vi "SDSU_DACS.vi"(0 "refnum":i32, 5 "Command":string, 7 "physical unit":string, 9 "swhitches":string[](array[string]), 11 "error in (no error)":errorcluster, 12 "switch arguments":string[](array[string])) -> (4 "refnum out":i32, 6 "response":string, 15 "error out":errorcluster)   [LabVIEW 2016]
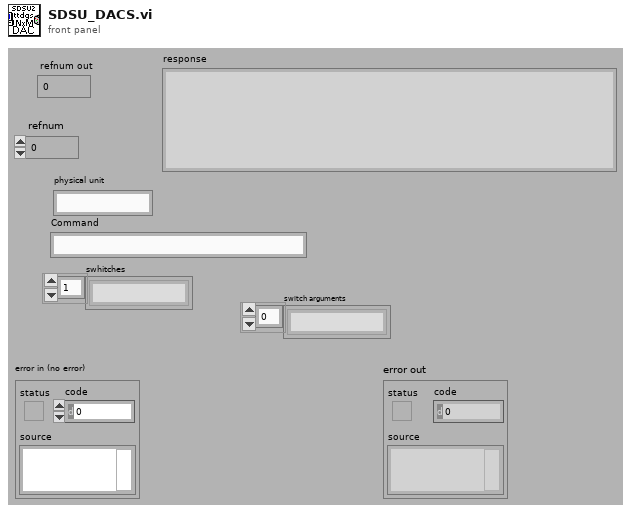
[diagram p1: front panel]
types:
  T1 = enum16{"read from file", "find", "set", "set_to_default", "get all"}
  T2 = enum16{"read from file", "find", "set", "set_to_default"}
  T3 = enum16{"read from file", "find", "set", "set_to_default", "get all", "resend_last"}
  T4 = typedef "CMN_ContStatus.ctl" = cluster{"Response":string, "power":bool, "shutter":bool, "artifdata":bool, "idlemode":bool, "reset":bool, "gain":u8, "speed":u8, "resetPCI":bool, "autoshutter":bool, "TempSetPoint":i32, "multipleextensions":bool, "displayImage":bool, "coadding":bool, "images being coadded":i32, "Operation Mode":enum16{"normal", "coadd", "fawler"}, "frames to write":cluster{"subs":bool, "reset":bool, "exposed":bool}, "fawler samples":i32, "write auto":bool, "datatype":string, "frames to display":cluster{"subs":bool, "reset":bool, "exposed":bool}, "sur":i32, "autoclear":bool}
  T5 = enum16{"Idle", "Exposing", "Paused", "AbortExp", "Reading", "AbortRead", "FinishedReading", "Resetting", "Reducing", "Initializing"}
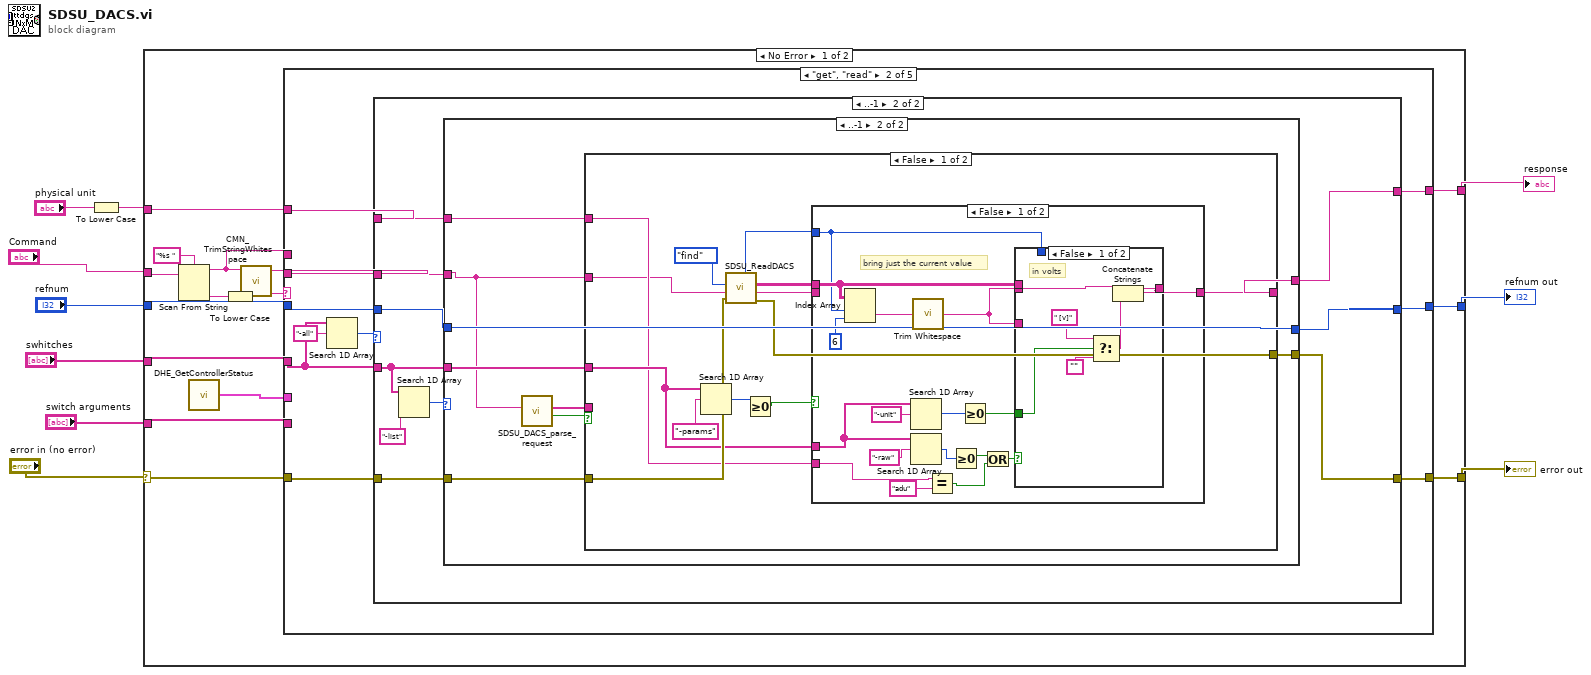
[diagram p0: block diagram]
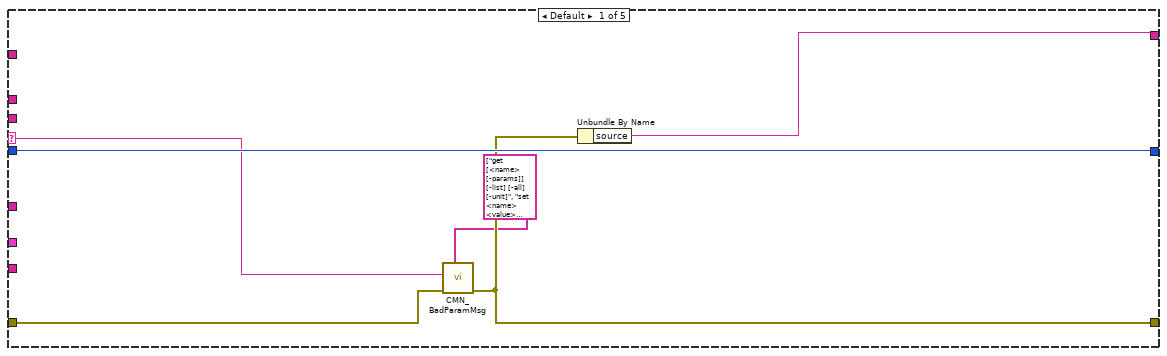
[diagram p2: hidden frame]
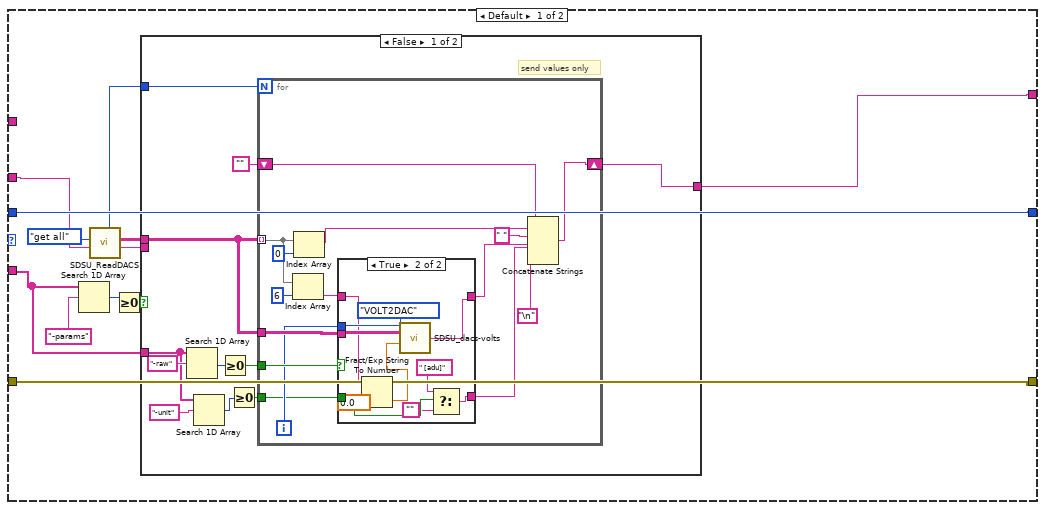
[diagram p3: hidden frame]
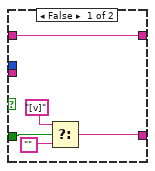
[diagram p4: hidden frame]
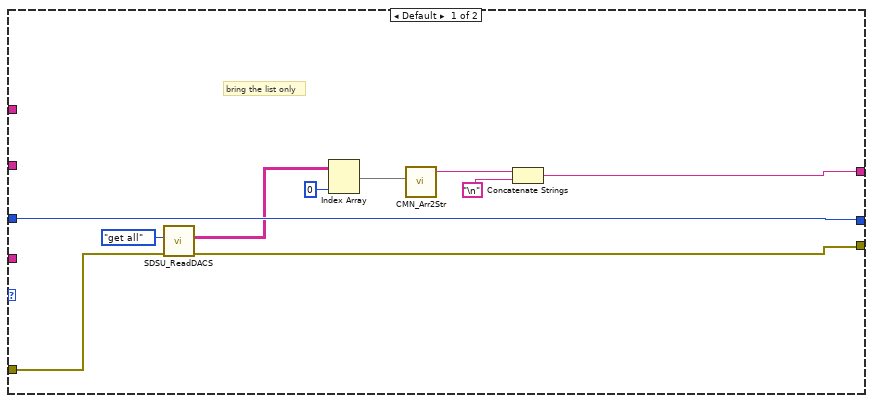
[diagram p6: hidden frame]
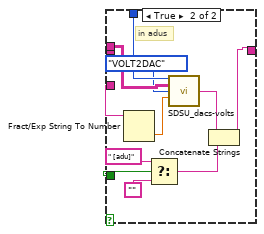
[diagram p7: hidden frame]
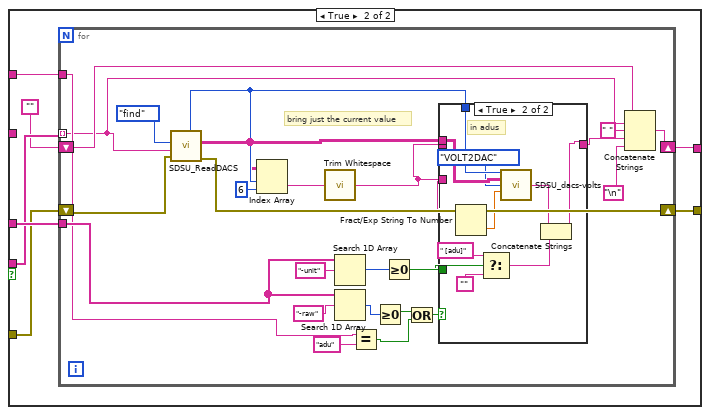
[diagram p9: hidden frame]
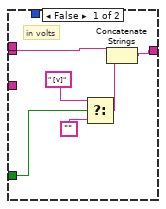
[diagram p10: hidden frame]
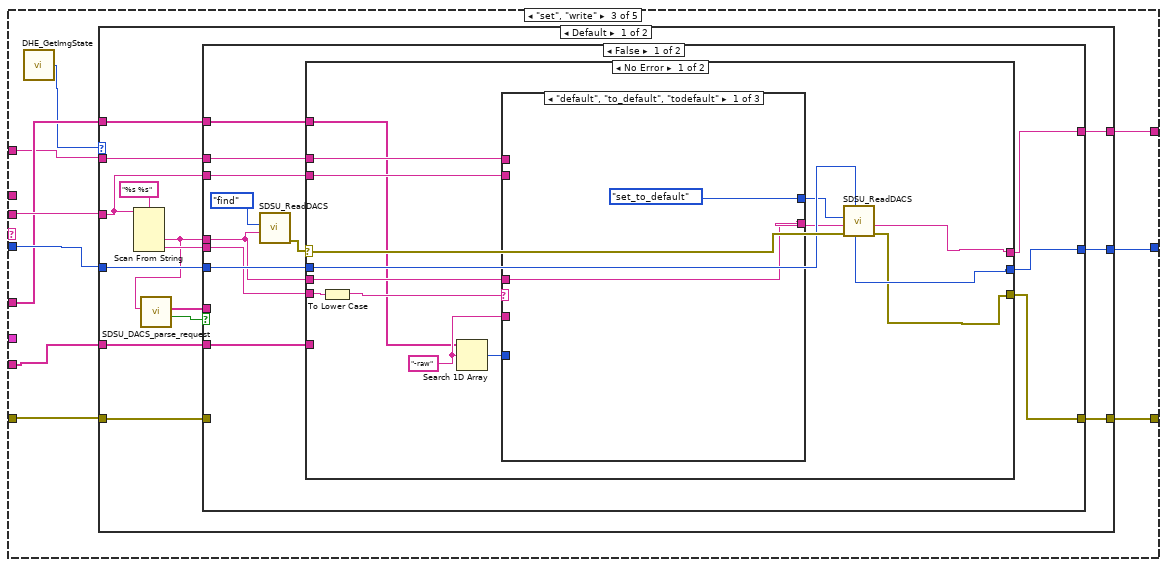
[diagram p11: hidden frame]
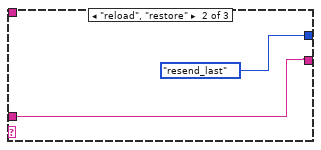
[diagram p12: hidden frame]
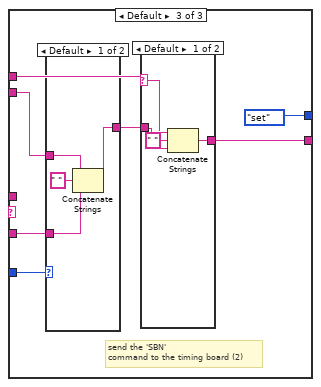
[diagram p13: hidden frame]
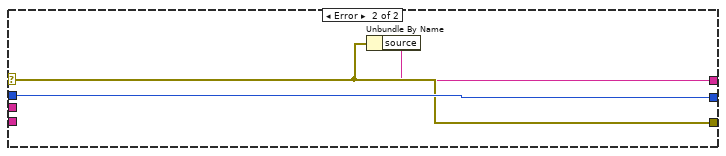
[diagram p16: hidden frame]
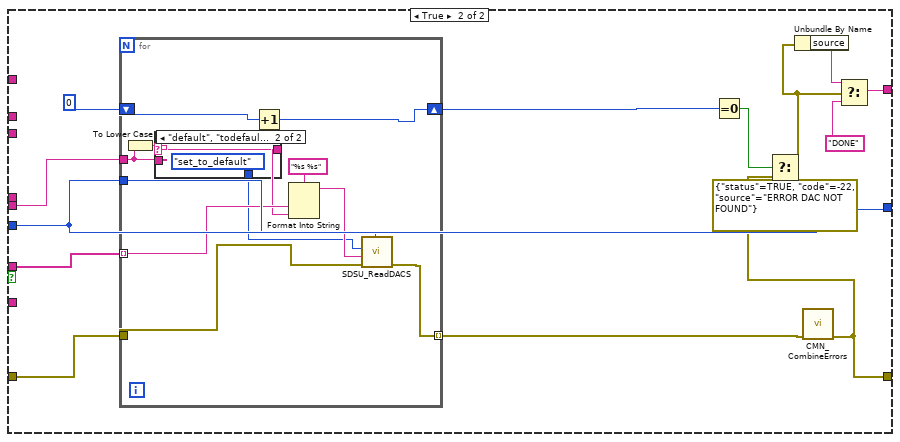
[diagram p17: hidden frame]
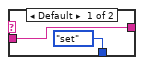
[diagram p18: hidden frame]
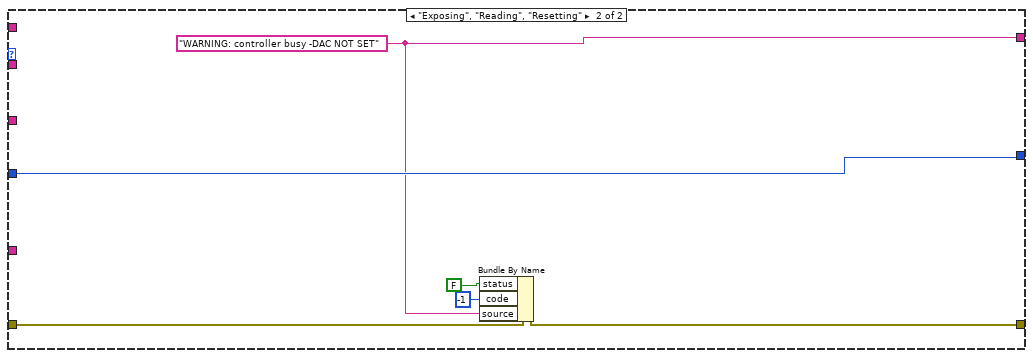
[diagram p19: hidden frame]
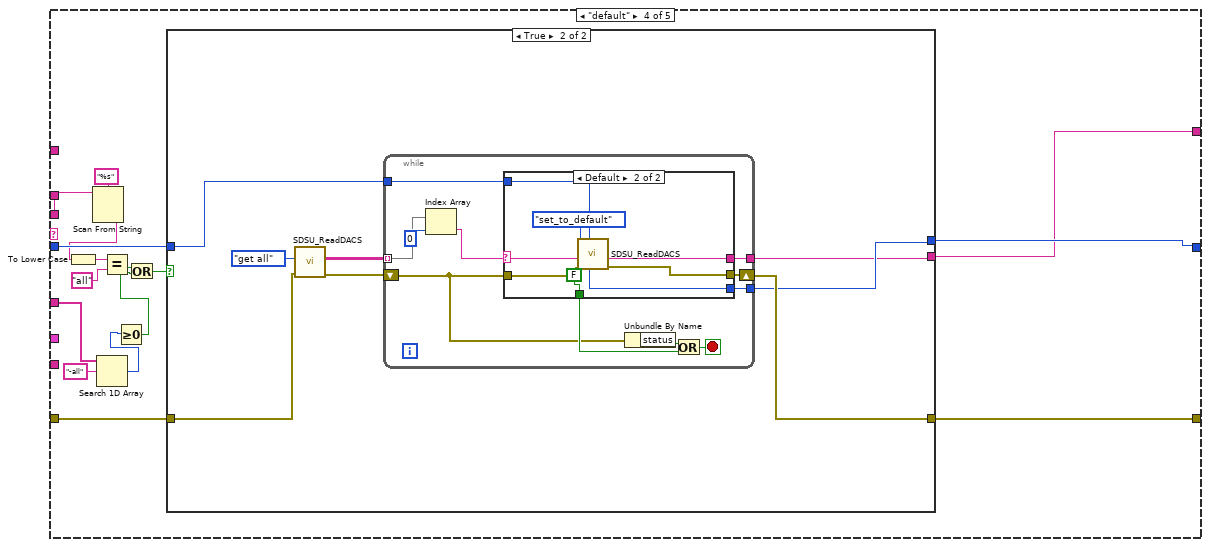
[diagram p20: hidden frame]
diagram:
  n1 = To Lower Case(string="physical unit") -> (all lower case string=w5:string)
  n2 = case shown="No Error" "error in (no error)" {
    selector: "error in (no error)" -> [w12 w440]
    tunnel: [w25 w440] -> w8
    tunnel: "refnum" -> [w24 w442]
    tunnel: [w23 w442] -> w10
    tunnel: "Command" -> [w16 _]
    tunnel: w5 -> [w15 _]
    tunnel: [w14 w441] -> w4
    tunnel: "swhitches" -> [w13 _]
    tunnel: "switch arguments" -> [w11 _]
    frame No Error {
      n3 = Scan From String(format string="%s " ("Format String"), input string=w16) -> (remaining string=w18:string, output 1=w19:string)  [unwired: 2 in, 3 out]
      n4 = call "DHE_GetControllerStatus.vi"() -> ("ControllerStatus"=w17:T4)  [unwired: 11 out]
      n5 = To Lower Case(string=w19) -> (all lower case string=w20:string)
      n6 = call "CMN_TrimStringWhitespace.vi"("string"=w18) -> ("trimmed string"=w21:string)  [unwired: 1 in, 8 out]
      n7 = case shown="\"get\", \"read\"" w20 {
        selector: w20 -> [w29 _ _ _ _]
        tunnel: w12 -> [w30 w36 w231 w338 w391]
        tunnel: [w28 w35 w229 w337 w390] -> w25
        tunnel: w24 -> [w31 w37 w227 w349 w402]
        tunnel: [w31 w41 w230 w336 w389] -> w23
        tunnel: w21 -> [_ w38 w232 w344 w397]
        tunnel: w17 -> [_ _ _ _ _]
        tunnel: w18 -> [_ _ _ _ _]
        tunnel: w15 -> [_ w39 w225 _ _]
        tunnel: [w27 w40 w228 w335 w388] -> w14
        tunnel: w13 -> [_ w34 w226 w334 w387]
        tunnel: w11 -> [_ _ w224 _ _]
        frame Default {
          n8 = call "CMN_BadParamMsg.vi"("valid params"=string[] ["get [<name> [-params]] [-list] [-all] [-unit]", "set <name> <value> [-raw] [default]", "default [-all]"], "error in (no error)"=w30, "parameter"=w29) -> ("error out"=w28:errorcluster)  [unwired: 1 in, 7 out]
          n9 = Unbundle By Name(w28) -> ("source"=w27:string)
        }
        frame "get", "read" {
          n10 = Search 1D Array(1D array=w34, element="-all") -> (index of element=w32:i32)  [unwired: 1 out]
          n11 = case shown="..-1" w32 {
            tunnel: [w50 w106] -> w41
            tunnel: [w51 w105] -> w40
            tunnel: w39 -> [_ w104]
            tunnel: w38 -> [w48 w103]
            tunnel: w37 -> [w50 w102]
            tunnel: w34 -> [w42 w99]
            tunnel: w36 -> [w43 w101]
            tunnel: [w43 w100] -> w35
            frame Default {
              n12 = Search 1D Array(1D array=w42, element="-params") -> (index of element=w52:i32)  [unwired: 1 out]
              n13 = call "SDSU_ReadDACS.vi"("argument"=w48, "action"=T1."get all") -> ("response"=w46:string, "Table"=w45:string[][], "index"=w44:i32)  [unwired: 3 in, 4 out]
              n14 = Greater Or Equal To 0?(x=w52) -> (x >= 0?=w47:bool)
              n15 = case shown="False" w47 {
                tunnel: [w62 w96] -> w51
                tunnel: w46 -> [_ w96]
                tunnel: w45 -> [w58 _]
                tunnel: w44 -> [w64 _]
                tunnel: w42 -> [w57 _]
                frame False {
                  # "send values only"
                  n16 = Search 1D Array(1D array=w57, element="-raw") -> (index of element=w60:i32)  [unwired: 1 out]
                  n17 = Search 1D Array(1D array=w57, element="-unit") -> (index of element=w55:i32)  [unwired: 1 out]
                  n18 = Greater Or Equal To 0?(x=w60) -> (x >= 0?=w59:bool)
                  n19 = Greater Or Equal To 0?(x=w55) -> (x >= 0?=w54:bool)
                  n20 = for {
                    N: w64 -> [_]
                    shift-right: [w79] -> w62
                    shift-left: "" -> [w78]
                    tunnel: w58 -> [w77] mode=indexing
                    tunnel: w59 -> [w71]
                    tunnel: w58 -> [w67]
                    tunnel: w54 -> [w65]
                    i -> [w66]
                    n21 = Index Array(array=w77, index=6) -> (element=w70:string)
                    n22 = Index Array(array=w77, index=0) -> (element=w74:string)
                    n23 = case shown="True" w71 {
                      tunnel: w70 -> [w84 w92]
                      tunnel: [w84 w90] -> w69
                      tunnel: [w80 w86] -> w68
                      tunnel: w67 -> [_ w95]
                      tunnel: w66 -> [_ w94]
                      tunnel: w65 -> [w83 w89]
                      frame False {
                        n24 = Select(t="[v]" ("string"), s=w83, f="") -> (s? t:f=w80:string)
                      }
                      frame True {
                        n25 = Fract/Exp String To Number(string=w92, default (0 dbl)=0.0) -> (number=w91:dbl)  [unwired: 3 out]
                        n26 = call "SDSU_dacs-volts.vi"("dac"=w94, "Table In"=w95, "action"=enum16{"DAC2VOLT", "VOLT2DAC"}."VOLT2DAC", "input value"=w91) -> ("string value"=w90:string)  [unwired: 11 out]
                        n27 = Select(t=" [adu]" ("string"), s=w89, f="") -> (s? t:f=w86:string)
                      }
                    }
                    n28 = Concatenate Strings(w78, w74, " " ("string"), w69, w68, "\n") -> (w79:string)
                  }
                }
                frame True {
                  # "send all the info"
                }
              }
            }
            frame ..-1 {
              n29 = Search 1D Array(1D array=w99, element="-list") -> (index of element=w97:i32)  [unwired: 1 out]
              n30 = case shown="..-1" w97 {
                tunnel: [w113 w125] -> w106
                tunnel: [w108 w122] -> w105
                tunnel: w104 -> [_ w120]
                tunnel: w103 -> [_ w119]
                tunnel: w102 -> [w113 w125]
                tunnel: w99 -> [_ w121]
                tunnel: w101 -> [w115 w124]
                tunnel: [w114 w123] -> w100
                frame Default {
                  # "bring the list only"
                  n31 = call "SDSU_ReadDACS.vi"("error in (no error)"=w115, "action"=T1."get all") -> ("error out"=w114:errorcluster, "Table"=w112:string[][])  [unwired: 3 in, 5 out]
                  n32 = Index Array(array=w112, index (col)=0 ("disabled index (col)")) -> (element=w110:string[])  [unwired: 1 in]
                  n33 = call "CMN_Arr2Str.vi"("Array in"=w110) -> ("string out"=w109:string)  [unwired: 10 out]
                  n34 = Concatenate Strings(w109, "\n") -> (w108:string)
                }
                frame ..-1 {
                  n35 = call "SDSU_DACS_parse_request.vi"("desired points"=w119) -> ("mult. points?"=w118:bool, "names"=w117:string[])  [unwired: 9 out]
                  n36 = case shown="False" w118 {
                    tunnel: w124 -> [w137 w176]
                    tunnel: [w136 w177] -> w123
                    tunnel: [w131 w175] -> w122
                    tunnel: w121 -> [w130 w180]
                    tunnel: w120 -> [w127 w179]
                    tunnel: w119 -> [w126 _]
                    tunnel: w117 -> [_ w178]
                    frame False {
                      n37 = Search 1D Array(1D array=w130, element="-params") -> (index of element=w134:i32)  [unwired: 1 out]
                      n38 = call "SDSU_ReadDACS.vi"("error in (no error)"=w137, "argument"=w126, "action"=T2."find") -> ("error out"=w136:errorcluster, "response"=w132:string, "Table"=w128:string[][], "index"=w129:i32)  [unwired: 2 in, 3 out]
                      n39 = Greater Or Equal To 0?(x=w134) -> (x >= 0?=w133:bool)
                      n40 = case shown="False" w133 {
                        tunnel: w132 -> [_ w173]
                        tunnel: [w153 w173] -> w131
                        tunnel: w130 -> [w152 _]
                        tunnel: w129 -> [w142 _]
                        tunnel: w128 -> [w143 _]
                        tunnel: w127 -> [w148 _]
                        frame False {
                          # "bring just the current value"
                          n41 = Index Array(array=w143, index (row)=w142, index (col)=6 ("line index")) -> (element=w140:string)
                          n42 = Search 1D Array(1D array=w152, element="-unit") -> (index of element=w150:i32)  [unwired: 1 out]
                          n43 = Search 1D Array(1D array=w152, element="-raw") -> (index of element=w154:i32)  [unwired: 1 out]
                          n44 = call <vilib>:"Trim Whitespace.vi"("string"=w140) -> ("trimmed string"=w139:string)  [unwired: 1 in]
                          n45 = Equal?(x=w148, y="adu") -> (x = y?=w144:bool)
                          n46 = Greater Or Equal To 0?(x=w154) -> (x >= 0?=w145:bool)
                          n47 = Greater Or Equal To 0?(x=w150) -> (x >= 0?=w149:bool)
                          n48 = Or(x=w145, y=w144) -> (x .or. y?=w146:bool)
                          n49 = case shown="False" w146 {
                            tunnel: w139 -> [w161 _]
                            tunnel: [w160 w166] -> w153
                            tunnel: w142 -> [_ w172]
                            tunnel: w143 -> [_ w171]
                            tunnel: w139 -> [_ w169]
                            tunnel: w149 -> [w157 w165]
                            frame False {
                              # "in volts"
                              n50 = Select(t=" [v]" ("string"), s=w157, f="") -> (s? t:f=w156:string)
                              n51 = Concatenate Strings(w161, w156) -> (w160:string)
                            }
                            frame True {
                              # "in adus"
                              n52 = Fract/Exp String To Number(string=w169) -> (number=w168:dbl)  [unwired: 4 out]
                              n53 = Select(t=" [adu]" ("string"), s=w165, f="") -> (s? t:f=w162:string)
                              n54 = call "SDSU_dacs-volts.vi"("dac"=w172, "Table In"=w171, "action"=enum16{"DAC2VOLT", "VOLT2DAC"}."VOLT2DAC", "input value"=w168) -> ("string value"=w167:string)  [unwired: 11 out]
                              n55 = Concatenate Strings(w167, w162) -> (w166:string)
                            }
                          }
                        }
                        frame True {
                          # "bring the parameters"
                        }
                      }
                    }
                    frame True {
                      n56 = for {
                        tunnel: w180 -> [w204]
                        tunnel: w179 -> [w203]
                        tunnel: w178 -> [w189] mode=indexing
                        shift-right: [w202] -> w177
                        shift-left: w176 -> [w201]
                        shift-right: [w191] -> w175
                        shift-left: "" -> [w190]
                        # "bring just the current value"
                        n57 = call "SDSU_ReadDACS.vi"("error in (no error)"=w201, "argument"=w189, "action"=T2."find") -> ("error out"=w202:errorcluster, "Table"=w182:string[][], "index"=w185:i32)  [unwired: 2 in, 4 out]
                        n58 = Index Array(array=w182, index (row)=w185, index (col)=6 ("disabled index (col)")) -> (element=w181:string)
                        n59 = call <vilib>:"Trim Whitespace.vi"("string"=w181) -> ("trimmed string"=w183:string)  [unwired: 1 in]
                        n60 = Search 1D Array(1D array=w204, element="-unit") -> (index of element=w197:i32)  [unwired: 1 out]
                        n61 = Search 1D Array(1D array=w204, element="-raw") -> (index of element=w199:i32)  [unwired: 1 out]
                        n62 = Equal?(x=w203, y="adu") -> (x = y?=w192:bool)
                        n63 = Greater Or Equal To 0?(x=w199) -> (x >= 0?=w193:bool)
                        n64 = Greater Or Equal To 0?(x=w197) -> (x >= 0?=w196:bool)
                        n65 = Or(x=w193, y=w192) -> (x .or. y?=w194:bool)
                        n66 = case shown="True" w194 {
                          tunnel: w183 -> [w211 _]
                          tunnel: [w210 w216] -> w187
                          tunnel: w185 -> [_ w222]
                          tunnel: w182 -> [_ w221]
                          tunnel: w183 -> [_ w219]
                          tunnel: w196 -> [w207 w215]
                          frame False {
                            # "in volts"
                            n67 = Select(t=" [v]" ("string"), s=w207, f="") -> (s? t:f=w206:string)
                            n68 = Concatenate Strings(w211, w206) -> (w210:string)
                          }
                          frame True {
                            # "in adus"
                            n69 = Fract/Exp String To Number(string=w219) -> (number=w218:dbl)  [unwired: 4 out]
                            n70 = Select(t=" [adu]" ("string"), s=w215, f="") -> (s? t:f=w212:string)
                            n71 = call "SDSU_dacs-volts.vi"("dac"=w222, "Table In"=w221, "action"=enum16{"DAC2VOLT", "VOLT2DAC"}."VOLT2DAC", "input value"=w218) -> ("string value"=w217:string)  [unwired: 11 out]
                            n72 = Concatenate Strings(w217, w212) -> (w216:string)
                          }
                        }
                        n73 = Concatenate Strings(w190, w189, " " ("string"), w187, "\n") -> (w191:string)
                      }
                    }
                  }
                }
              }
            }
          }
        }
        frame "set", "write" {
          n74 = call "DHE_GetImgState.vi"() -> ("DHE_ImgState"=w223:T5)  [unwired: 9 out]
          n75 = case shown="Default" w223 {
            tunnel: w232 -> [w239 _]
            tunnel: w231 -> [w236 w332]
            tunnel: [w246 w333] -> w230
            tunnel: [w245 w329] -> w229
            tunnel: [w244 w328] -> w228
            tunnel: w227 -> [w243 w333]
            tunnel: w226 -> [w242 _]
            tunnel: w225 -> [w241 _]
            tunnel: w224 -> [w238 _]
            frame Default {
              n76 = Scan From String(format string="%s %s", input string=w239) -> (output 1=w235:string, output 2=w237:string)  [unwired: 2 in, 5 out]
              n77 = call "SDSU_DACS_parse_request.vi"("desired points"=w235) -> ("mult. points?"=w234:bool, "names"=w233:string[])  [unwired: 9 out]
              n78 = case shown="False" w234 {
                tunnel: [w258 w305] -> w246
                tunnel: [w257 w302] -> w245
                tunnel: [w256 w308] -> w244
                tunnel: w243 -> [w255 w305]
                tunnel: w242 -> [w254 _]
                tunnel: w241 -> [w253 _]
                tunnel: w239 -> [w252 _]
                tunnel: w237 -> [w251 w311]
                tunnel: w235 -> [w249 _]
                tunnel: w238 -> [w247 _]
                tunnel: w236 -> [_ w307]
                tunnel: w233 -> [_ w298]
                frame False {
                  n79 = call "SDSU_ReadDACS.vi"("argument"=w249, "action"=enum16{"read from file", "find", "set"}."find") -> ("error out"=w248:errorcluster)  [unwired: 3 in, 6 out]
                  n80 = case shown="No Error" w248 {
                    selector: w248 -> [w272 w296]
                    tunnel: w255 -> [w271 w297]
                    tunnel: [w270 w297] -> w258
                    tunnel: [w269 w296] -> w257
                    tunnel: [w268 w295] -> w256
                    tunnel: w254 -> [w259 _]
                    tunnel: w253 -> [w266 _]
                    tunnel: w252 -> [w273 _]
                    tunnel: w251 -> [w267 _]
                    tunnel: w249 -> [w260 _]
                    tunnel: w247 -> [_ _]
                    frame No Error {
                      w264 = "-raw" ("element")
                      n81 = To Lower Case(string=w267) -> (all lower case string=w262:string)
                      n82 = Search 1D Array(1D array=w259, element=w264) -> (index of element=w265:i32)  [unwired: 1 out]
                      n83 = case shown="\"default\", \"to_default\", \"todefault\"" w262 {
                        tunnel: w273 -> [_ _ w284]
                        tunnel: w266 -> [_ _ w283]
                        tunnel: w265 -> [_ _ w282]
                        tunnel: w264 -> [_ _ w281]
                        tunnel: [w275 w277 w279] -> w263
                        tunnel: [T3."set_to_default" ("action") T3."resend_last" ("action") T2."set" ("action")] -> w261
                        tunnel: w260 -> [w275 w277 _]
                        frame "default", "to_default", "todefault" {
                        }
                        frame "reload", "restore" {
                        }
                        frame Default {
                          # "send the 'SBN'\ncommand to the timing board (2)"
                          n84 = case shown="Default" w282 {
                            tunnel: w284 -> [w293 w294]
                            tunnel: w281 -> [w291 _]
                            tunnel: [w290 w294] -> w280
                            frame Default {
                              n85 = Concatenate Strings(w293, " " ("string"), w291) -> (w290:string)
                            }
                            frame ..-1 {
                            }
                          }
                          n86 = case shown="Default" w283 {
                            selector: w283 -> [w286 _]
                            tunnel: w280 -> [w288 w289]
                            tunnel: [w285 w289] -> w279
                            frame Default {
                              n87 = Concatenate Strings(w288, " " ("string"), w286) -> (w285:string)
                            }
                            frame "", " " {
                            }
                          }
                        }
                      }
                      n88 = call "SDSU_ReadDACS.vi"("fd"=w271, "error in (no error)"=w272, "argument"=w263, "action"=w261) -> ("error out"=w269:errorcluster, "response"=w268:string, "fd out"=w270:i32)  [unwired: 1 in, 4 out]
                    }
                    frame Error {
                      n89 = Unbundle By Name(w296) -> ("source"=w295:string)
                    }
                  }
                }
                frame True {
                  n90 = for {
                    tunnel: w311 -> [w313]
                    tunnel: w307 -> [w323]
                    tunnel: [w322] -> w306 mode=indexing
                    tunnel: w305 -> [w321]
                    shift-right: [w319] -> w303
                    shift-left: 0 -> [w320]
                    tunnel: w298 -> [w316] mode=indexing
                    n91 = To Lower Case(string=w313) -> (all lower case string=w315:string)
                    n92 = case shown="\"default\", \"todefault\"" w315 {
                      selector: w315 -> [_ w327]
                      tunnel: [w325 w327] -> w314
                      tunnel: w313 -> [w325 _]
                      tunnel: [T1."set" ("action") T1."set_to_default" ("action")] -> w312
                      frame Default {
                      }
                      frame "default", "todefault" {
                      }
                    }
                    n93 = Increment(x=w320) -> (x+1=w319:i32)
                    n94 = Format Into String(format string="%s %s", w316, w314) -> (resulting string=w317:string)  [unwired: 2 in, 1 out]
                    n95 = call "SDSU_ReadDACS.vi"("fd"=w321, "error in (no error)"=w323, "argument"=w317, "action"=w312) -> ("error out"=w322:errorcluster)  [unwired: 1 in, 6 out]
                  }
                  n96 = Equal To 0?(x=w303) -> (x = 0?=w301:bool)
                  n97 = call "CMN_CombineErrors.vi"("Errors"=w306) -> ("error out"=w302:errorcluster)  [unwired: 10 out]
                  n98 = Select(t=errorcluster {"status"=TRUE, "code"=-22, "source"="ERROR DAC NOT FOUND"}, s=w301, f=w302) -> (s? t:f=w300:errorcluster)
                  n99 = Unbundle By Name(w300) -> ("source"=w309:string)
                  n100 = Select(t=w309, s=w300, f="DONE") -> (s? t:f=w308:string)
                }
              }
            }
            frame "Exposing", "Reading", "Resetting" {
              w328 = "WARNING: controller busy -DAC NOT SET" ("source")
              n101 = Bundle By Name(cluster=w332, "status"=FALSE, "code"=-1, "source"=w328) -> (w329:errorcluster)
            }
          }
        }
        frame "default" {
          n102 = Scan From String(format string="%s", input string=w344) -> (output 1=w341:string)  [unwired: 2 in, 4 out]
          n103 = To Lower Case(string=w341) -> (all lower case string=w340:string)
          n104 = Search 1D Array(1D array=w334, element="-all") -> (index of element=w347:i32)  [unwired: 1 out]
          n105 = Equal?(x=w340, y="all") -> (x = y?=w342:bool)
          n106 = Greater Or Equal To 0?(x=w347) -> (x >= 0?=w346:bool)
          n107 = Or(x=w342, y=w346) -> (x .or. y?=w345:bool)
          n108 = case shown="True" w345 {
            tunnel: w349 -> [w351 w360]
            tunnel: w338 -> [w355 w363]
            tunnel: [w354 w361] -> w337
            tunnel: [w351 w359] -> w336
            tunnel: [w350 w358] -> w335
            frame False {
              w350 = "ERROR: unknown command" ("source")
              n109 = Bundle By Name(cluster=w355, "status"=TRUE, "code"=-22, "source"=w350) -> (w354:errorcluster)
            }
            frame True {
              n110 = call "SDSU_ReadDACS.vi"("error in (no error)"=w363, "action"=T3."get all") -> ("error out"=w362:errorcluster, "Table"=w357:string[][])  [unwired: 3 in, 5 out]
              n111 = while {
                tunnel: w357 -> [w367] mode=indexing
                shift-right: [w368] -> w361
                shift-left: w362 -> [w364]
                tunnel: w360 -> [w373]
                tunnel: [w372] -> w359
                tunnel: [w371] -> w358
                stop <- w370 stop-if-true
                n112 = Index Array(array=w367, index=0 ("disabled index (col)")) -> (element=w366:string)
                n113 = case shown="Default" w366 {
                  selector: w366 -> [_ w380]
                  tunnel: w364 -> [w378 w385]
                  tunnel: w373 -> [w375 w384]
                  tunnel: [w375 w383] -> w372
                  tunnel: ["OK" ("response") w382] -> w371
                  tunnel: [w378 w381] -> w368
                  tunnel: [TRUE FALSE] -> w365
                  frame "", " " {
                  }
                  frame Default {
                    n114 = call "SDSU_ReadDACS.vi"("fd"=w384, "error in (no error)"=w385, "argument"=w380, "action"=T1."set_to_default") -> ("error out"=w381:errorcluster, "response"=w382:string, "fd out"=w383:i32)  [unwired: 1 in, 4 out]
                  }
                }
                n115 = Unbundle By Name(w364) -> ("status"=w369:bool)
                n116 = Or(x=w369, y=w365) -> (x .or. y?=w370:bool)
              }
            }
          }
        }
        frame "last", "reload", "restore", "set_last" {
          n117 = Scan From String(format string="%s", input string=w397) -> (output 1=w394:string)  [unwired: 2 in, 4 out]
          n118 = To Lower Case(string=w394) -> (all lower case string=w393:string)
          n119 = Search 1D Array(1D array=w387, element="-all") -> (index of element=w400:i32)  [unwired: 1 out]
          n120 = Equal?(x=w393, y="all") -> (x = y?=w395:bool)
          n121 = Greater Or Equal To 0?(x=w400) -> (x >= 0?=w399:bool)
          n122 = Or(x=w395, y=w399) -> (x .or. y?=w398:bool)
          n123 = case shown="True" w398 {
            tunnel: w402 -> [w404 w412]
            tunnel: w391 -> [w408 w415]
            tunnel: [w407 w413] -> w390
            tunnel: [w404 w411] -> w389
            tunnel: [w403 w410] -> w388
            frame False {
              w403 = "ERROR: unknown command" ("source")
              n124 = Bundle By Name(cluster=w408, "status"=TRUE, "code"=-22, "source"=w403) -> (w407:errorcluster)
            }
            frame True {
              n125 = call "SDSU_ReadDACS.vi"("error in (no error)"=w415, "action"=T1."get all") -> ("error out"=w414:errorcluster, "Table"=w409:string[][])  [unwired: 3 in, 5 out]
              n126 = while {
                tunnel: w409 -> [w420] mode=indexing
                shift-right: [w421] -> w413
                shift-left: w414 -> [w417]
                tunnel: w412 -> [w426]
                tunnel: [w425] -> w411
                tunnel: [w424] -> w410
                stop <- w423 stop-if-true
                n127 = Index Array(array=w420, index=0 ("disabled index (col)")) -> (element=w419:string)
                n128 = case shown="Default" w419 {
                  selector: w419 -> [_ w434]
                  tunnel: w417 -> [w431 w439]
                  tunnel: w426 -> [w428 w438]
                  tunnel: [w428 w437] -> w425
                  tunnel: ["OK" ("response") w436] -> w424
                  tunnel: [w431 w435] -> w421
                  tunnel: [TRUE FALSE] -> w418
                  frame "", " " {
                  }
                  frame Default {
                    n129 = call "SDSU_ReadDACS.vi"("fd"=w438, "error in (no error)"=w439, "argument"=w434, "action"=T3."resend_last") -> ("error out"=w435:errorcluster, "response"=w436:string, "fd out"=w437:i32)  [unwired: 1 in, 4 out]
                  }
                }
                n130 = Unbundle By Name(w417) -> ("status"=w422:bool)
                n131 = Or(x=w422, y=w418) -> (x .or. y?=w423:bool)
              }
            }
          }
        }
      }
    }
    frame Error {
      n132 = Unbundle By Name(w440) -> ("source"=w441:string)  [unwired: 1 out]
    }
  }
  "refnum out" <- w10
  "error out" <- w8
  "response" <- w4
